vi "LVClass_WavefrontCorrectorSet Get Parameter Option.vi"(0 "WavefrontCorrectorSet in":refnum<class "WavefrontCorrectorSet.lvclass">, 5 "parameter_name":string, 11 "error in (no error)":errorcluster) -> (3 "Settable-Gettable?":cluster{"Settable":bool, "Gettable":bool}, 4 "WavefrontCorrectorSet out":refnum<class "WavefrontCorrectorSet.lvclass">, 6 "DefaultValueExist":bool, 8 "minmax":bool, 10 "String enum":bool, 14 "Settable-Gettable on fly?":cluster{"Settable":bool, "Gettable":bool}, 15 "error out":errorcluster)   [LabVIEW 2020, in "WavefrontCorrectorSet.lvclass"]
doc: "WavefrontCorrector parameter options getter given its name which should have\nbeen read with Imop_WavefrontCorrectorSet_GetParameterName.\n\n--------------------------------------------------------------------------------\n\n<B>wavefrontcorrector_setIn </B> : WavefrontCorrectorSet object.\n<B>wavefrontcorrector_setOut </B> : WavefrontCorrectorSet object.\n<B>parameter_name </B> : Parameter name.\n<B>is_settable </B> : Parameter value is writeable.\n<B>is_gettable </B> : Parameter value is readable.\n<B>has_default_value </B> : Parameter has a default value.\n<B>has_limits </B> : If parameter is a number, its value is to be selected between a min and a max\n value.\n<B>is_string_enum </B> : If parameter is a string, its value is to be selected in a finite set of\n values.\n<B>is_settable_on_fly </B> : Parameter is writeable while wavefront corrector is running, and a value\n change is taken into account asap.\n<B>is_gettable_on_fly </B> : Parameter is readable while wavefront correcto is running, and the return\n value will be the one currently used.\n<B>ErrorIn </B> : Error\n<B>ErrorOut </B> : Error\n\n--------------------------------------------------------------------------------"
uses:
  WavefrontCorrectorSet.lvclass
  WavefrontCorrectorSet.lvclass/WavefrontCorrectorSet.ctl
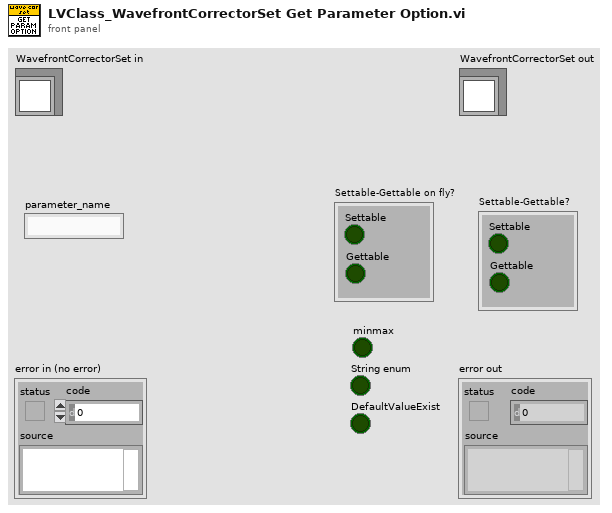
[diagram p1: front panel]
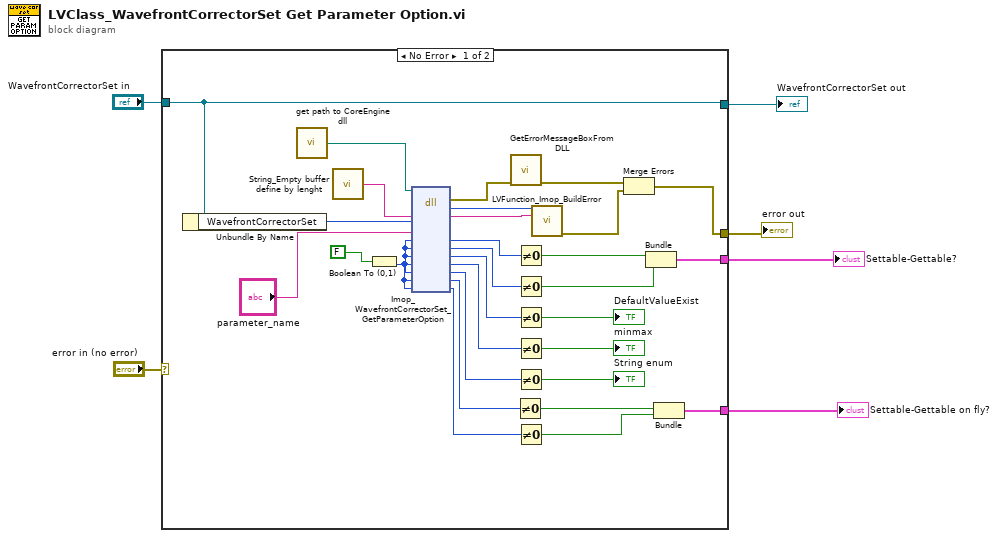
[diagram p0: block diagram]
diagram:
  n1 = case shown="No Error" "error in (no error)" {
    selector: "error in (no error)" -> [_ w36]
    tunnel: "WavefrontCorrectorSet in" -> [w20 w37]
    tunnel: [w20 w37] -> w3
    tunnel: [w16 w36] -> w4
    tunnel: [w14 _] -> w6
    tunnel: [w7 _] -> w5
    frame No Error {
      n2 = Unbundle By Name(w20) -> ("WavefrontCorrectorSet"=w19:i32)
      n3 = call "get path to CoreEngine dll.vi"() -> ("path to c_interface_vc100.dll"=w31:path)  [unwired: 12 in, 3 out]
      n4 = call "String_Empty buffer define by lenght.vi"() -> ("Empty buffer"=w33:string)  [unwired: 1 in]
      n5 = Boolean To (0,1)(Boolean=FALSE) -> (0, 1=w10:i16)
      n6 = dll-call lib="D:/soft/HASO_v3/C_interface/Sources/Build/vc100/Release/c_interface_vc100.dll" fn="Imop_WavefrontCorrectorSet_GetParameterOption"(path in=w31, "message"=w33, "objet"=w19, "parameter_name"="parameter_name", "Settable"=w10, "Gettable"=w10, "DefaultValueExist"=w10, "minmax"=w10, "StringEnum"=w10, "Settable_onfly"=w10, "Gettable_onfly"=w10) -> (error out=w30:errorcluster, "return type"=w35:i32, "message"=w34:string, "Settable"=w28:u8, "Gettable"=w27:u8, "DefaultValueExist"=w26:u8, "minmax"=w24:u8, "StringEnum"=w22:u8, "Settable_onfly"=w12:u8, "Gettable_onfly"=w11:u8)  [unwired: 4 in, 1 out]
      n7 = call "GetErrorMessageBoxFromDLL.vi"("error IN"=w30) -> ("error OUT"=w18:errorcluster)  [unwired: 10 in]
      n8 = Not Equal To 0?(x=w12) -> (x != 0?=w9:bool)
      n9 = Not Equal To 0?(x=w28) -> (x != 0?=w15:bool)
      n10 = Not Equal To 0?(x=w27) -> (x != 0?=w13:bool)
      n11 = Not Equal To 0?(x=w26) -> (x != 0?=→"DefaultValueExist":bool)
      n12 = Not Equal To 0?(x=w24) -> (x != 0?=→"minmax":bool)
      n13 = Not Equal To 0?(x=w22) -> (x != 0?=→"String enum":bool)
      n14 = Not Equal To 0?(x=w11) -> (x != 0?=w8:bool)
      n15 = call "LVFunction_Imop_BuildError.vi"("code"=w35, "String to Prepend to source (\"\")"=w34) -> ("error out"=w17:errorcluster)  [unwired: 13 in]
      n16 = Merge Errors(w18, w17) -> (w16:errorcluster)
      n17 = Bundle(w15, w13) -> (w14:cluster{bool, bool})  [unwired: 1 in]
      n18 = Bundle(w9, w8) -> (w7:cluster{bool, bool})  [unwired: 1 in]
    }
    frame Error {
    }
  }
  "error out" <- w4
  "WavefrontCorrectorSet out" <- w3
  "Settable-Gettable?" <- w6
  "Settable-Gettable on fly?" <- w5
